vi "Get IP Address.vi"() -> (3 "IP Address":string)   [LabVIEW 2016, in "Assert API Components.lvlib" / "Log Assert Core.lvlib"]
doc: "Gets the IP Address of the system the vi is run on (PC or RT Target)"
uses:
  Log Assert Core.lvlib
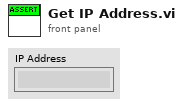
[diagram p1: front panel]
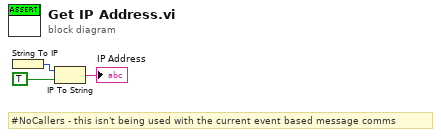
[diagram p0: block diagram]
diagram:
  # "#NoCallers - this isn't being used with the current event based message comms"
  n1 = String To IP() -> (0:w3:u32)  [unwired: 1 in]
  n2 = IP To String(1:TRUE ("dot notation? (F)"), 2:w3) -> (0:→"IP Address":string)
